vi "PlayerRead.vi"(9 "NXT":T1={"Hardware"="NXT", "Flattened String"=""}) -> (0 "Completed":bool, 1 "Powers":i16[](array[numeric]), 3 "NXT":T1={"Hardware"="NXT", "Flattened String"=""})   [LabVIEW 2010, in "Player.lvlib"]
uses:
  Player.lvlib
  <vilib>/NXT/Subs/LVHSConnector.ctl
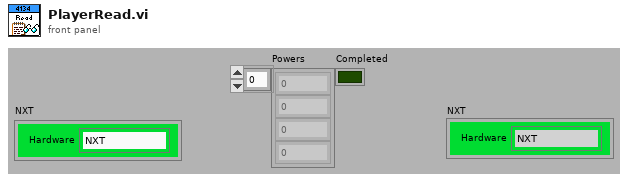
[diagram p1: front panel]
types:
  T1 = typedef "LVHSConnector.ctl" = cluster{"Hardware":string, "Flattened String":string}
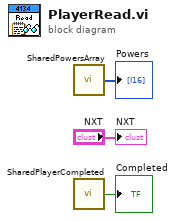
[diagram p0: block diagram]
diagram:
  n1 = call "SharedPowersArray.vi"() -> ("Powers"=→"Powers":i16[])  [unwired: 2 in]
  n2 = call "SharedPlayerCompleted.vi"() -> ("PlayerCompleted"=→"Completed":bool)  [unwired: 2 in]
  "NXT" <- "NXT"
